vi "Receive Command Response.vi"(0 "connection ID":refnum<k5>, 9 "Timeout (60000ms)":i32=60000, 11 "error in (no error)":errorcluster) -> (4 "connection ID out":refnum<k5>, 6 "OK Packet Metadata":T2 {"Server Status" format="%.0x"}, 15 "error out":errorcluster)   [LabVIEW 2014, in "hse-db.lvlib" / "MySQL (TCP).lvlib"]
uses:
  MySQL (TCP).lvlib
  Controls/OK Packet Metadata.ctl
  Controls/Return Packet Types.ctl
panel:
  out "Array":T1[](array[typedef])
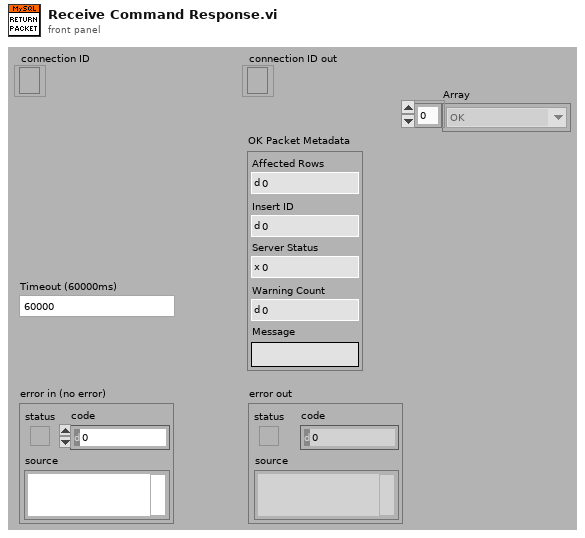
[diagram p1: front panel]
types:
  T1 = typedef "hse-db.lvlib/MySQL (TCP).lvlib/Return Packet Types.ctl" = enum16{"OK", "Result Set Header", "Error", "Field", "Row", "EOF"}
  T2 = typedef "hse-db.lvlib/MySQL (TCP).lvlib/OK Packet Metadata.ctl" = cluster{"Affected Rows":u64, "Insert ID":u64, "Server Status":u16, "Warning Count":u16, "Message":string}
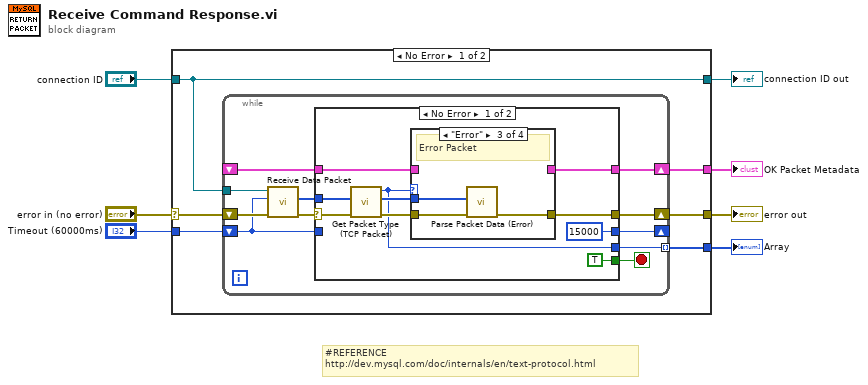
[diagram p0: block diagram]
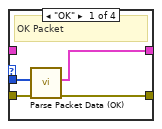
[diagram p2: hidden frame]
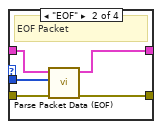
[diagram p3: hidden frame]
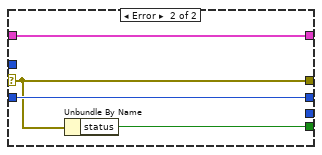
[diagram p5: hidden frame]
diagram:
  # "#REFERENCE\nhttp://dev.mysql.com/doc/internals/en/text-protocol.html"
  n1 = case shown="No Error" "error in (no error)" {
    selector: "error in (no error)" -> [w11 w53]
    tunnel: [w13 _] -> w5
    tunnel: [w12 w53] -> w7
    tunnel: "connection ID" -> [w8 w52]
    tunnel: [w8 w52] -> w3
    tunnel: "Timeout (60000ms)" -> [w10 _]
    tunnel: [w9 _] -> w1
    frame No Error {
      n2 = while {
        shift-right: [w23] -> w12
        shift-left: w11 -> [w22]
        shift-right: [w24] -> w13
        shift-left: _ -> [w19]
        tunnel: [w17] -> w9 mode=indexing
        shift-right: [w16] -> _
        shift-left: w10 -> [w15]
        tunnel: w8 -> [w14]
        stop <- w20 stop-if-true
        n3 = call "Receive Data Packet.vi"("error in"=w22, "Timeout (60000ms)"=w15, "connection ID"=w14) -> ("error out"=w18:errorcluster, "TCP/IP Data"=w21:u8[])  [unwired: 5 in, 2 out]
        n4 = case shown="No Error" w18 {
          selector: w18 -> [w30 w48]
          tunnel: [w34 w51] -> w24
          tunnel: [w33 w48] -> w23
          tunnel: w21 -> [w31 _]
          tunnel: [TRUE ("status") w50] -> w20
          tunnel: w19 -> [w32 w51]
          tunnel: [w27 _] -> w17
          tunnel: [15000 ("Timeout (60000ms)") w49] -> w16
          tunnel: w15 -> [_ w49]
          frame No Error {
            n5 = call "Get Packet Type (TCP Packet).vi"("Error In"=w30, "TCP/IP Data in"=w31) -> ("Error Out"=w29:errorcluster, "TCP/IP Data out"=w28:u8[], "Return Packet Type"=w27:T1)  [unwired: 7 in]
            n6 = case shown="\"Error\"" w27 {
              tunnel: w28 -> [w38 w41 w44 _]
              tunnel: [w35 w42 _ _] -> w34
              tunnel: w29 -> [w37 w40 w46 w47]
              tunnel: [w36 w39 w45 w47] -> w33
              tunnel: w32 -> [_ w43 _ _]
              frame "OK" {
                # "OK Packet"
                n7 = call "Parse Packet Data (OK).vi"("Error In"=w37, "Recieved Bytes"=w38) -> ("Error Out"=w36:errorcluster, "Packet Metadata out"=w35:T2)  [unwired: 8 in]
              }
              frame "EOF" {
                # "EOF Packet"
                n8 = call "Parse Packet Data (EOF).vi"("Error In"=w40, "Recieved Bytes"=w41, "Packet Metadata In"=w43) -> ("Error Out"=w39:errorcluster, "Packet Metadata Out"=w42:T2)  [unwired: 7 in]
              }
              frame "Error" {
                # "Error Packet"
                n9 = call "Parse Packet Data (Error).vi"("error in (no error)"=w46, "Recieved Bytes"=w44) -> ("error out"=w45:errorcluster)  [unwired: 9 in]
              }
              frame Default {
              }
            }
          }
          frame Error {
            n10 = Unbundle By Name(w48) -> ("status"=w50:bool)
          }
        }
      }
    }
    frame Error {
    }
  }
  "error out" <- w7
  "OK Packet Metadata" <- w5
  "connection ID out" <- w3
  "Array" <- w1
